vi "Abeles Brewster Analysis.vi"(0 "Open Substrate File":path, 1 "Open Film File":path, 2 "q Starting":dbl, 3 "q Final":dbl, 4 "Do AB Analysis":bool, 5 "calculate error":bool, 6 "Error (degrees)":dbl) -> (10 "ángulo B valor medio":dbl, 11 "IR Película 2":dbl format="%#.4g", 12 "Film qB +error":dbl, 13 "Film RI +error":dbl format="%#.4g", 14 "Substrate qB":dbl, 15 "Film qB":dbl, 16 "Substrate RI":dbl format="%#.4g", 17 "Film RI":dbl format="%#.4g", 19 "Curves":cluster{dbl[], dbl[]}[](graph))   [LabVIEW 2025, in "Control de MaP.lvlib"]
uses:
  Control de MaP.lvlib
panel:
  out "otros ángulos cero":dbl[](array[numeric])
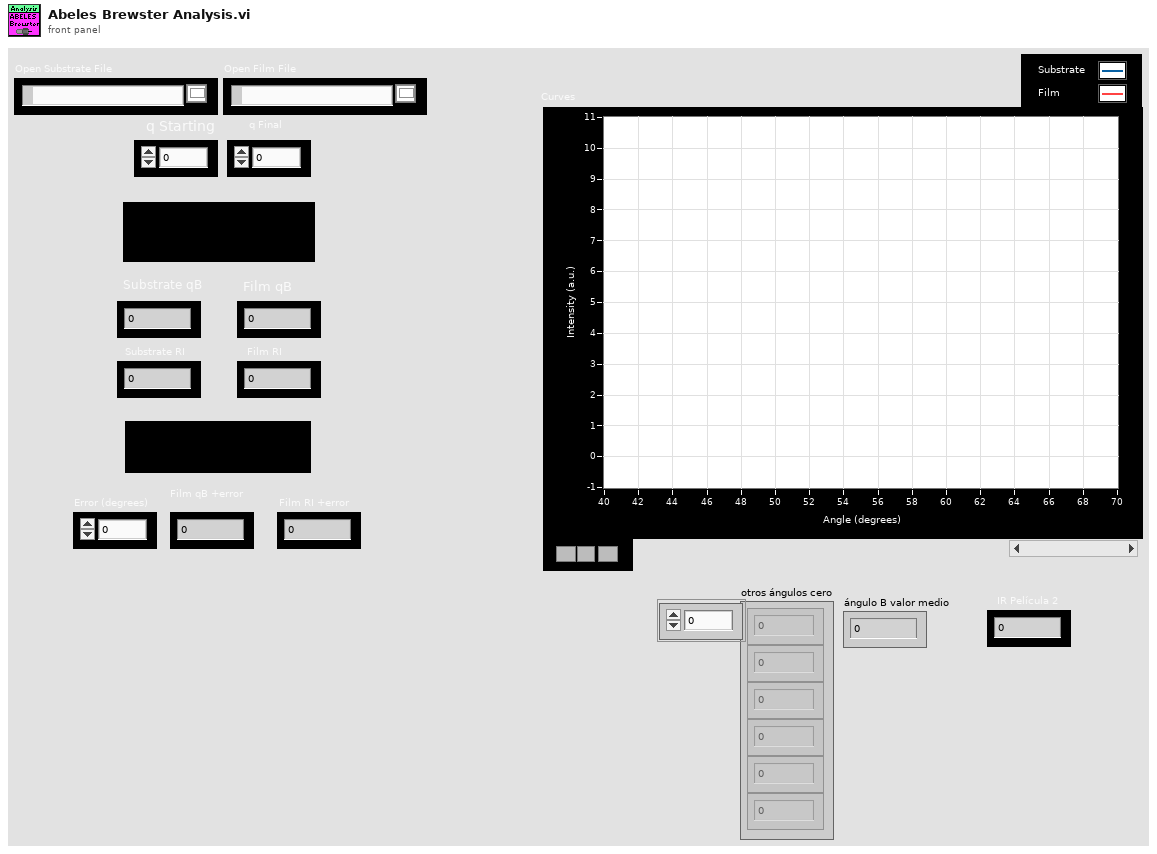
[diagram p1: front panel]
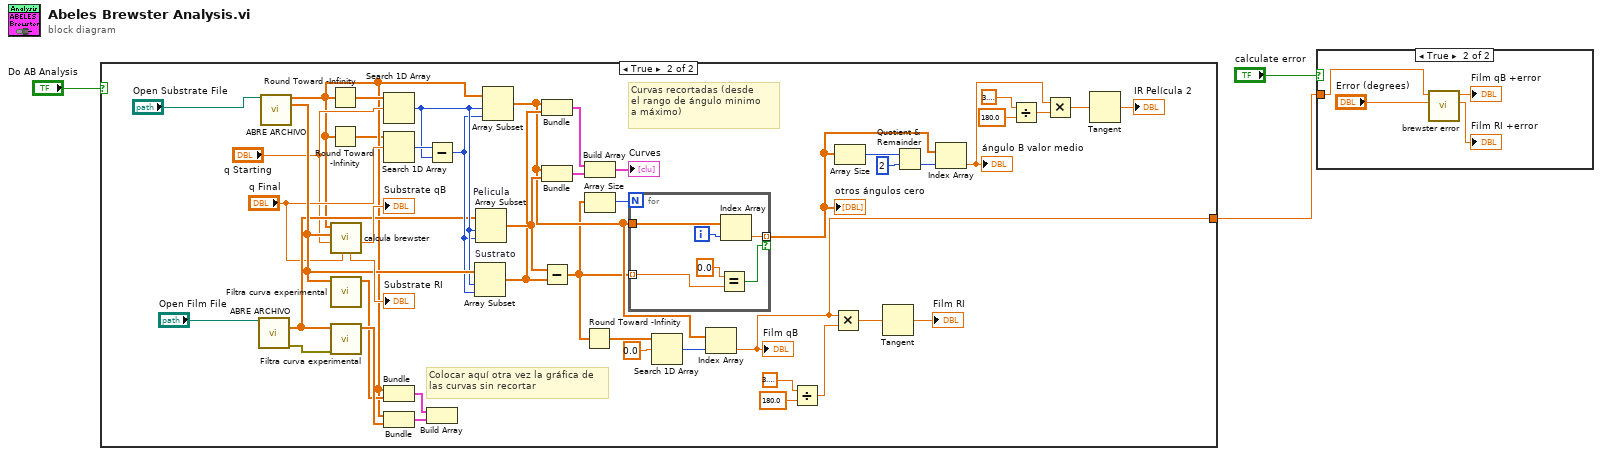
[diagram p0: block diagram]
diagram:
  n1 = case shown="True" "Do AB Analysis" {
    tunnel: [_ w28] -> w2
    frame False {
    }
    frame True {
      # "Curvas recortadas (desde\nel rango de ángulo minimo \na máximo)"
      # "Colocar aquí otra vez la gráfica de\nlas curvas sin recortar"
      n2 = call "ABRE ARCHIVO.vi"("File Path Control"="Open Film File") -> ("EJE Y"=w11:dbl[], "error out"=w45:errorcluster)  [unwired: 9 in, 4 out]
      n3 = call "ABRE ARCHIVO.vi"("File Path Control"="Open Substrate File") -> ("EJE X"=w7:dbl[], "EJE Y"=w32:dbl[])  [unwired: 9 in, 4 out]
      n4 = Round Toward -Infinity(1:w7) -> (0:w8:dbl[])
      n5 = Round Toward -Infinity(1:w7) -> (0:w6:dbl[])
      n6 = call "calcula brewster.vi"("Ángulo Final"="q Final", "Ángulo Inicial"="q Starting", "EJE Y"=w32, "EJE X"=w7) -> ("Ángulo de Brewster"=→"Substrate qB":dbl, "Índice de Refracción"=→"Substrate RI":dbl)  [unwired: 3 in, 3 out]
      n7 = call "Filtra curva experimental.vi"("Y"=w32) -> ("Y Filtrada"=w23:dbl[])  [unwired: 8 in, 2 out]
      n8 = call "Filtra curva experimental.vi"("error in (no error)"=w45, "Y"=w11) -> ("Y Filtrada"=w24:dbl[])  [unwired: 7 in, 2 out]
      n9 = Search 1D Array(1D array=w8, element="q Starting") -> (index of element=w26:i32)  [unwired: 1 in]
      n10 = Search 1D Array(1D array=w6, element="q Final") -> (index of element=w44:i32)  [unwired: 1 in]
      n11 = Bundle("EJE X"=w7, "Y Filtrada"=w23) -> (w40:cluster{"EJE X":dbl[], "Y Filtrada":dbl[]})  [unwired: 1 in]
      n12 = Bundle("EJE X"=w7, "Y Filtrada"=w24) -> (w41:cluster{"EJE X":dbl[], "Y Filtrada":dbl[]})  [unwired: 1 in]
      n13 = Subtract(x=w44, y=w26) -> (x-y=w25:i32)
      n14 = Build Array(w40, w41) -> ()  [unwired: 1 out]
      n15 = Array Subset "Sustrato"(array=w32, index=w26, length=w25) -> (w30:dbl[])
      n16 = Array Subset "Pelicula"(array=w11, index=w26, length=w25) -> (w31:dbl[])
      n17 = Array Subset(array=w7, index=w26, length=w25) -> (w22:dbl[])
      n18 = Bundle(w22, w30) -> (w29:cluster{dbl[], dbl[]})  [unwired: 1 in]
      n19 = Bundle(w22, w31) -> (w43:cluster{dbl[], dbl[]})  [unwired: 1 in]
      n20 = Subtract(x=w31, y=w30) -> (x-y=w4:dbl[])
      n21 = Round Toward -Infinity(1:w4) -> (0:w5:dbl[])
      n22 = Build Array(w29, w43) -> (→"Curves":cluster{dbl[], dbl[]}[])
      n23 = Array Size(array=w4) -> (size(s)=w27:i32)
      n24 = for {
        N: w27 -> [_]
        tunnel: w4 -> [w55] mode=indexing
        tunnel: [w50] -> w19 mode=indexing if=w53
        tunnel: w22 -> [w52]
        i -> [w51]
        n25 = Equal?(x=0.0, y=w55) -> (x = y?=w53:bool)
        n26 = Index Array(array=w52, index=w51) -> (element=w50:dbl)
      }
      "otros ángulos cero" <- w19
      n27 = Search 1D Array(1D array=w5, element=0.0) -> (index of element=w38:i32)  [unwired: 1 in]
      n28 = Index Array(array=w22, index=w38) -> (element=w28:dbl)
      "Film qB" <- w28
      n29 = Divide(x=3.141592653589793, y=180.0) -> (x/y=w35:dbl)
      n30 = Multiply(x=w28, y=w35) -> (x*y=w36:dbl)
      n31 = Array Size(array=w19) -> (size(s)=w21:i32)
      n32 = Tangent(1:w36) -> (0:→"Film RI":dbl)
      n33 = Quotient & Remainder(x=w21, y=2) -> (floor(x/y)=w12:i32)  [unwired: 1 out]
      n34 = Index Array(array=w19, index=w12) -> (element=w15:dbl)
      "ángulo B valor medio" <- w15
      n35 = Divide(x=3.141592653589793, y=180.0) -> (x/y=w18:dbl)
      n36 = Multiply(x=w15, y=w18) -> (x*y=w13:dbl)
      n37 = Tangent(1:w13) -> (0:→"IR Película 2":dbl)
    }
  }
  n38 = case shown="True" "calculate error" {
    tunnel: w2 -> [_ w58]
    frame False {
    }
    frame True {
      n39 = call "brewster error.vi"("Error (grados)"="Error (degrees)", "Numeric Control"=w58) -> ("Índice de Refracción +error"=→"Film RI +error":dbl, "Ángulo de Brewster +error"=→"Film qB +error":dbl)  [unwired: 8 in]
    }
  }
